vi "integer to 7-seg decoder.vi"(0 "Integer number":u16, 2 "Display On/Off":bool, 3 "dp":bool, 5 "Is negative? (F)":bool) -> (7 "7-seg digit":T1)   [LabVIEW 2015]
doc: "This module converts any integer between 0 and 9 to its equivalent on a 7-segment display, and has a separate input for turning on the decimal point (dp). This is the normal operating state. On the other hand, as a second state, it has an independent input to indicate a minus sign (turns on the segment g). Finally, it has a complete shutdown of the display, and this state has priority over all others."
uses:
  controls/green 7-seg display.ctl
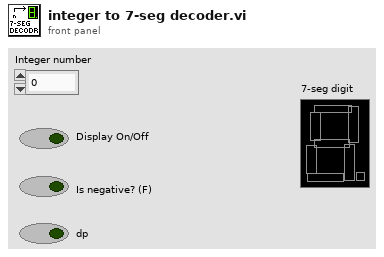
[diagram p1: front panel]
types:
  T1 = typedef "green 7-seg display.ctl" = cluster{"a-seg":bool, "b-seg":bool, "c-seg":bool, "d-seg":bool, "e-seg":bool, "f-seg":bool, "g-seg":bool, "dp-seg":bool}
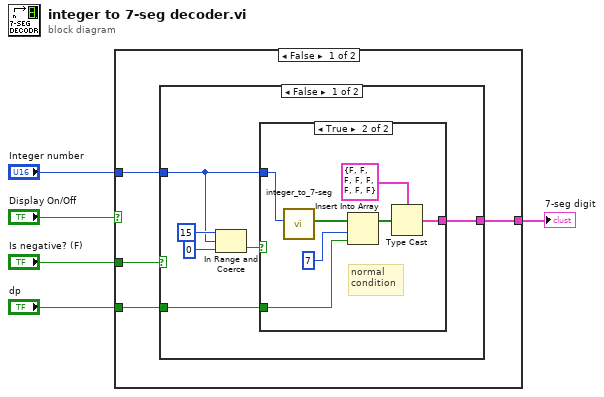
[diagram p0: block diagram]
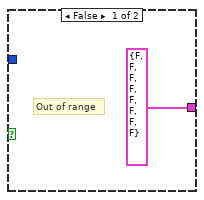
[diagram p2: hidden frame]
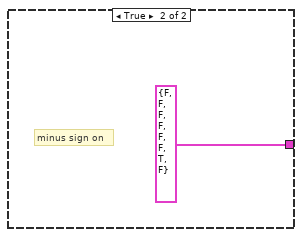
[diagram p3: hidden frame]
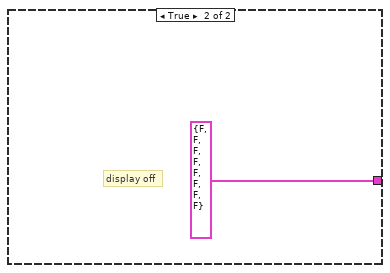
[diagram p4: hidden frame]
diagram:
  n1 = case shown="False" "Display On/Off" {
    tunnel: [w8 T1 {"a-seg"=FALSE, "b-seg"=FALSE, "c-seg"=FALSE, "d-seg"=FALSE, "e-seg"=FALSE, "f-seg"=FALSE, "g-seg"=FALSE, "dp-seg"=FALSE} ("7-seg digit")] -> w1
    tunnel: "Is negative? (F)" -> [w9 _]
    tunnel: "Integer number" -> [w7 _]
    tunnel: "dp" -> [w6 _]
    frame False {
      n2 = case shown="False" w9 {
        tunnel: [w12 T1 {"a-seg"=FALSE, "b-seg"=FALSE, "c-seg"=FALSE, "d-seg"=FALSE, "e-seg"=FALSE, "f-seg"=FALSE, "g-seg"=TRUE, "dp-seg"=FALSE} ("7-seg digit")] -> w8
        tunnel: w7 -> [w10 _]
        tunnel: w6 -> [w11 _]
        frame False {
          n3 = In Range and Coerce(upper limit=u16 15, x=w10, lower limit=u16 0) -> (In Range?=w13:bool)  [unwired: 1 out]
          n4 = case shown="True" w13 {
            tunnel: w10 -> [_ w21]
            tunnel: [T1 {"a-seg"=FALSE, "b-seg"=FALSE, "c-seg"=FALSE, "d-seg"=FALSE, "e-seg"=FALSE, "f-seg"=FALSE, "g-seg"=FALSE, "dp-seg"=FALSE} ("7-seg digit") w17] -> w12
            tunnel: w11 -> [_ w22]
            frame False {
              # "Out of range"
            }
            frame True {
              # "normal \ncondition"
              n5 = call "integer_to_7-seg.vi"("Entero"=w21) -> ("7-seg"=w20:bool[])  [unwired: 10 in]
              n6 = Insert Into Array(array=w20, index=7, new element=w22) -> (w19:bool[])
              n7 = Type Cast(type=T1 {"a-seg"=FALSE, "b-seg"=FALSE, "c-seg"=FALSE, "d-seg"=FALSE, "e-seg"=FALSE, "f-seg"=FALSE, "g-seg"=FALSE, "dp-seg"=FALSE} ("7-seg digit"), x=w19) -> (*(type *) &x=w17:T1)
            }
          }
        }
        frame True {
          # "minus sign on"
        }
      }
    }
    frame True {
      # "display off"
    }
  }
  "7-seg digit" <- w1
